vi "Automatic Image Scale.vi"(6 "Box":cluster{"width":sgl, "height":sgl}, 7 "Y offset (point)":sgl, 8 "error in (no error)":errorcluster, 9 "Scale percent IN":sgl, 10 "GetInstanceImage IN":refnum<k24>, 11 "Document":refnum<k24>) -> (0 "error out":errorcluster, 1 "Scale percent OUT":sgl, 2 "GetInstanceImage OUT":refnum<k24>, 3 "Document duplicate":refnum<k24>, 5 "Scaled Image width":sgl)   [LabVIEW 2013]
doc: "Version 1.0\nDeveloped by Jean-Marc Simard\nCopyright © 2010, Exaprom Inc.\nAll rights reserved.\nLicense: BSD\n\nWith iTextSharp 4.1.6 (http://itextsharp.sourceforge.net)\nunder Mozilla Public License Version 1.1\n(http://www.mozilla.org/MPL/MPL-1.1.html)"
uses:
  C:/Users/MaxCorp/Documents/GitHub/TopView/DLL/itextsharp.dll
  DLL/itextsharp.dll
  Controls/PDF Report Xcontrol/PDF Report.xctl
panel:
  in  "PDF Report":T21(xcontrol)
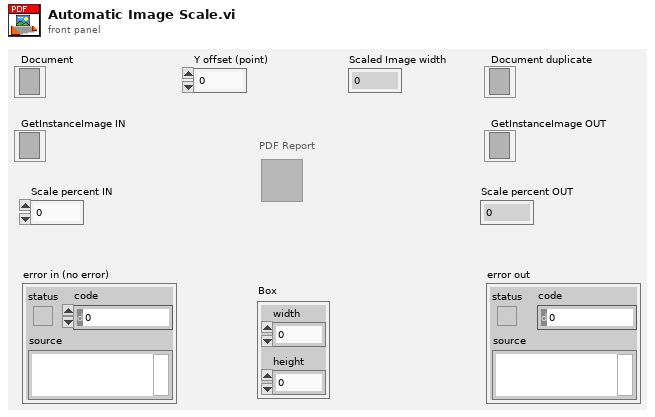
[diagram p1: front panel]
types:
  T1 = typedef "Font cluster.ctl" = cluster{"Name":string, "Size":T2, "Color":T3, "Style":cluster{"Bold":bool, "Italic":bool, "Underline":bool, "Strikeout":bool}}
  T2 = typedef "Font size.ctl" = sgl
  T3 = typedef "Font color.ctl" = u32
  T4 = typedef "Unit.ctl" = enum16{"inch", "mm"}
  T5 = typedef "Paragraphe cluster.ctl" = cluster{" Aligment":T6, "Line spacing":T7}
  T6 = typedef "Texte alignement.ctl" = enum16{"Select", "CENTER", "JUSTIFY", "LEFT", "RIGHT"}
  T7 = typedef "Line spacing.ctl" = enum16{"Select", "1.0", "1.5", "2.0"}
  T8 = typedef "Page dimensions.ctl" = cluster{"Start at page":i32, "Orientation":T9, "widht":sgl, "height":sgl, "Margin left":sgl, "Margin right":sgl, "Margin top":sgl, "Margin bottom":sgl}
  T9 = typedef "Page Orientation.ctl" = enum16{"Portrait", "Landscape"}
  T10 = typedef "Image or Table Caption.ctl" = cluster{"Caption":string, "Separator":string, "Position":enum16{"Above", "Below"}}
  T11 = typedef "Header Footer [ ].ctl" = T12[]
  T12 = typedef "Header Footer cluster.ctl" = cluster{"Start page":i32, "Type":T13, "Alignment":T14, "Vertical Alignement":T15, "Image (%)":sgl, "Page #":T16, "Text":string, "Path":string, "Font":T1, "Font refnum":refnum<k24>, "Line":cluster{"Line":T17, "Thickness (points)":sgl, "Colour":T3}}
  T13 = typedef "Header Footer Type.ctl" = enum16{"Select", "Text", "Text + hyperlink", "Page number", "Image", "Image + hyperlink"}
  T14 = typedef "Header footer horiz alignment.ctl" = enum16{"Left", "Center", "Right"}
  T15 = typedef "Cell Vertical alignment.ctl" = enum16{"TOP", "MIDDLE", "BOTTOM"}
  T16 = typedef "Page number.ctl" = cluster{"Text 1":string, "Text 2":string, "Text 3":string}
  T17 = typedef "Header Footer Line.ctl" = enum16{"No line", "Horizontal line"}
  T18 = typedef "Watermark cluster2.ctl" = cluster{"Show? (F)":bool, "Type":enum16{"Image", "Text"}, "Opacity (%)":sgl, "Rotate(°)":sgl, "Position":cluster{"Position":T19, "X":sgl, "Y":sgl}, "Image path":path, "Scaled(%)":sgl, "Image refnum":refnum<k24>, "Text":string, "Font":cluster{"Name":string, "Size":T2, "Color":T3}, "Font refnum":refnum<k24>, "Alignment":T14, "Automatic":bool}
  T19 = typedef "Watermark Position.ctl" = enum16{"Absolute", "Center (page)", "Center (text section)"}
  T20 = typedef "System Fonts.ctl" = cluster{"Font name [ ]":string[], "Font and file names [ ]":cluster{"Font name":string, "File name":string}[]}
  T21 = cluster{"Document":refnum<k24>, "Writer":refnum<k24>, "Default Font":refnum<k24>, "Default Font cluster":T1, "Path":path, "Unit (default = mm)":T4, "Paragraphe cluster":T5, "Pages dimensions [ ]":T8[], "Captions":cluster{"Image":T10, "Image counter":u16, "Table":T10, "Table counter":u16, "Font":T1}, "Header":T11, "Footer":T11, "Watermark ":T18, "Actual VI name":string, "System Fonts":T20}
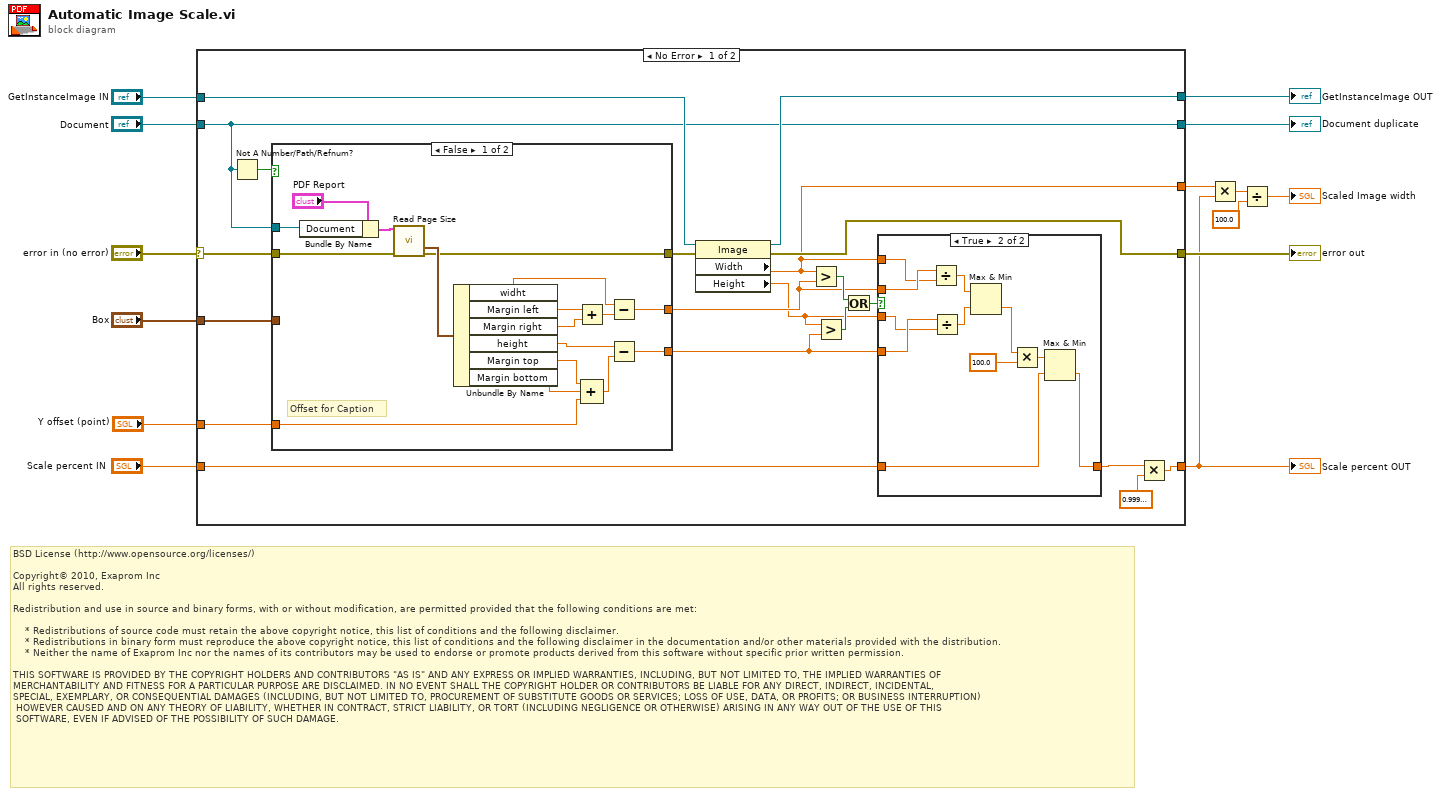
[diagram p0: block diagram]
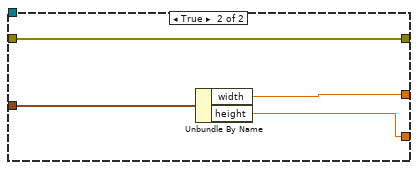
[diagram p2: hidden frame]
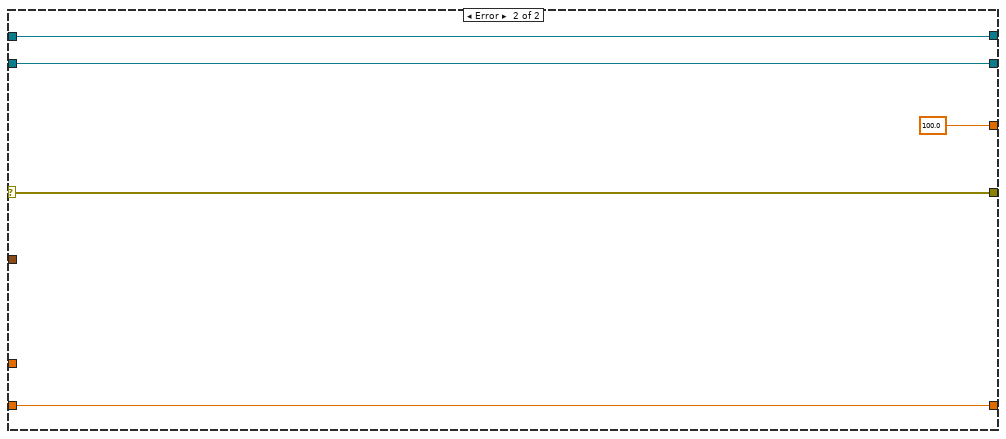
[diagram p4: hidden frame]
diagram:
  # "BSD License (http://www.opensource.org/licenses/)\n\nCopyright© 2010, Exaprom Inc\nAll rights reserved.\n\nRedistribution and use in source and binary forms, with or without modification, are permitted provided that the following conditions are met:\n\n    * Redistributions of source code must retain the above copyright notice, this list of conditions and the following disclaimer.\n    * Redistributions in binary form must reproduce the above copyright notice, this list of conditions and the following disclaimer in the documentation and/or other materials provided with the distribution.\n    * Neither the name of Exaprom Inc nor the names of its contributors may be used to endorse or promote products derived from this software without specific prior written permission.\n\nTHIS SOFTWARE IS PROVIDED BY THE COPYRIGHT HOLDERS AND CONTRIBUTORS \"AS IS\" AND ANY EXPRESS OR IMPLIED WARRANTIES, INCLUDING, BUT NOT LIMITED TO, THE IMPLIED WARRANTIES OF \nMERCHANTABILITY AND FITNESS FOR A PARTICULAR PURPOSE ARE DISCLAIMED. IN NO EVENT SHALL THE COPYRIGHT HOLDER OR CONTRIBUTORS BE LIABLE FOR ANY DIRECT, INDIRECT, INCIDENTAL,\nSPECIAL, EXEMPLARY, OR CONSEQUENTIAL DAMAGES (INCLUDING, BUT NOT LIMITED TO, PROCUREMENT OF SUBSTITUTE GOODS OR SERVICES; LOSS OF USE, DATA, OR PROFITS; OR BUSINESS INTERRUPTION)\n HOWEVER CAUSED AND ON ANY THEORY OF LIABILITY, WHETHER IN CONTRACT, STRICT LIABILITY, OR TORT (INCLUDING NEGLIGENCE OR OTHERWISE) ARISING IN ANY WAY OUT OF THE USE OF THIS\n SOFTWARE, EVEN IF ADVISED OF THE POSSIBILITY OF SUCH DAMAGE."
  n1 = case shown="No Error" "error in (no error)" {
    selector: "error in (no error)" -> [w23 w70]
    tunnel: "GetInstanceImage IN" -> [w34 w72]
    tunnel: "Scale percent IN" -> [w27 w69]
    tunnel: [w17 w69] -> w5
    tunnel: [w21 w71] -> w12
    tunnel: [w26 w72] -> w11
    tunnel: "Document" -> [w21 w71]
    tunnel: [w24 w70] -> w9
    tunnel: "Box" -> [w22 _]
    tunnel: [w20 sgl 100.0 ("Width")] -> w6
    tunnel: "Y offset (point)" -> [w18 _]
    frame No Error {
      n2 = Not A Number/Path/Refnum?(number/path/refnum=w21) -> (NaN/Path/Refnum?=w25:bool)
      n3 = case shown="False" w25 {
        tunnel: w21 -> [w47 _]
        tunnel: [w38 w55] -> w33
        tunnel: [w49 w53] -> w30
        tunnel: [w48 w52] -> w19
        tunnel: w23 -> [w46 w55]
        tunnel: w22 -> [_ w54]
        tunnel: w18 -> [w35 _]
        frame False {
          # "Offset for Caption"
          n4 = Bundle By Name(cluster="PDF Report", "Document"=w47) -> (w36:T21)
          n5 = call "Read Page Size.vi"("PDF Report"=w36, "error in (no error)"=w46) -> ("Page (points)"=w45:T8, "error out"=w38:errorcluster)  [unwired: 12 out]
          n6 = Unbundle By Name(w45) -> ("widht"=w39:sgl, "Margin left"=w40:sgl, "Margin right"=w41:sgl, "height"=w42:sgl, "Margin top"=w44:sgl, "Margin bottom"=w43:sgl)
          n7 = Add(x=w40, y=w41) -> (x+y=w51:sgl)
          n8 = Compound Arithmetic op=ADD(w44, w43, w35) -> (w50:sgl)
          n9 = Subtract(x=w39, y=w51) -> (x-y=w49:sgl)
          n10 = Subtract(x=w42, y=w50) -> (x-y=w48:sgl)
        }
        frame True {
          n11 = Unbundle By Name(w54) -> ("width"=w53:sgl, "height"=w52:sgl)
        }
      }
      n12 = property class="Image"(reference=w34, error in=w33) -> (reference out=w26:refnum<k24>, error out=w24:errorcluster, "Width"=w20:sgl, "Height"=w29:sgl)
      n13 = Greater?(x=w20, y=w30) -> (0:w31:bool)
      n14 = Greater?(x=w29, y=w19) -> (0:w32:bool)
      n15 = Or(x=w31, y=w32) -> (x .or. y?=w28:bool)
      n16 = case shown="True" w28 {
        tunnel: w20 -> [_ w66]
        tunnel: w30 -> [_ w67]
        tunnel: w29 -> [_ w64]
        tunnel: w19 -> [_ w65]
        tunnel: w27 -> [w56 w61]
        tunnel: [w56 w60] -> w16
        frame False {
        }
        frame True {
          n17 = Divide(x=w67, y=w66) -> (x/y=w63:sgl)
          n18 = Divide(x=w65, y=w64) -> (x/y=w62:sgl)
          n19 = Max & Min(x=w63, y=w62) -> (min(x,y)=w58:sgl)  [unwired: 1 out]
          n20 = Multiply(x=w58, y=sgl 100.0) -> (x*y=w59:sgl)
          n21 = Max & Min(x=w59, y=w61) -> (min(x,y)=w60:sgl)  [unwired: 1 out]
        }
      }
      n22 = Multiply(x=w16, y=sgl 0.999) -> (x*y=w17:sgl)
    }
    frame Error {
    }
  }
  "Scale percent OUT" <- w5
  "Document duplicate" <- w12
  "GetInstanceImage OUT" <- w11
  "error out" <- w9
  n23 = Multiply(x=w6, y=w5) -> (x*y=w4:sgl)
  n24 = Divide(x=w4, y=sgl 100.0) -> (x/y=→"Scaled Image width":sgl)
